vi "DrawBigDigit.vi"(6 "color":fxp<+,3,3>, 8 "error in (no error)":errorcluster, 9 "Digit":i32, 10 "Position":T1, 11 "Game in":refnum<class "Game.lvclass">) -> (0 "error out":errorcluster, 3 "Game out":refnum<class "Game.lvclass">)   [LabVIEW 2019, in "RT_Game.lvlib" / "Game.lvclass"]
uses:
  Game.lvclass
  Coordinate.ctl
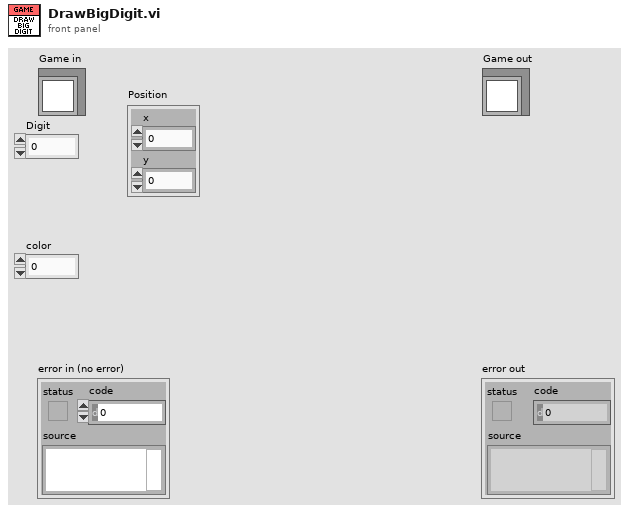
[diagram p1: front panel]
types:
  T1 = typedef "RT_Game.lvlib/Game.lvclass/Coordinate.ctl" = cluster{"x":dbl, "y":dbl}
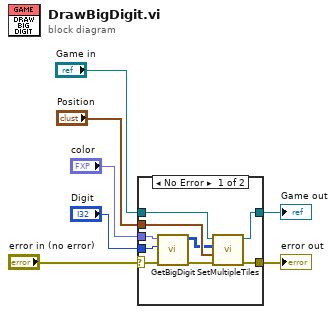
[diagram p0: block diagram]
diagram:
  n1 = case shown="No Error" "error in (no error)" {
    selector: "error in (no error)" -> [w16 w18]
    tunnel: [w15 w18] -> w6
    tunnel: [w14 w17] -> w4
    tunnel: "Game in" -> [w13 w17]
    tunnel: "Digit" -> [w12 _]
    tunnel: "Position" -> [w11 _]
    tunnel: "color" -> [w10 _]
    frame No Error {
      n2 = call "GetBigDigit.vi"("error in (no error)"=w16, "Digit"=w12, "color"=w10) -> ("error out"=w9:errorcluster, "Array"=w8:u32[][])  [unwired: 7 in]
      n3 = call "SetMultipleTiles.vi"("error in (no error)"=w9, "Position"=w11, "TileCodes"=w8, "Game in"=w13) -> ("error out"=w15:errorcluster, "Game out"=w14:refnum<class "Game.lvclass">)  [unwired: 6 in]
    }
    frame Error {
    }
  }
  "error out" <- w6
  "Game out" <- w4
